vi "Waveform CDB to power level.vi"(11 "Waveform CDB":waveform(cdb)) -> (3 "Power [Watt]":dbl)   [LabVIEW 2020]
uses:
  <vilib>/Analysis/5stat.llb/RMS (DBL).vi
  <vilib>/Analysis/NI_AALPro.lvlib
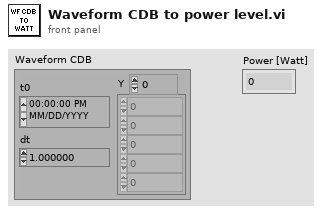
[diagram p1: front panel]
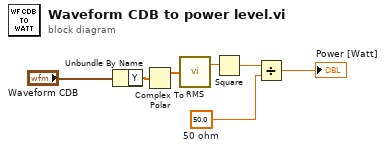
[diagram p0: block diagram]
diagram:
  w7 = 50.0  # 50 ohm
  n1 = Unbundle By Name("Waveform CDB") -> ("Y"=w5:cdb[])
  n2 = Complex To Polar(r * e^(i*theta)=w5) -> (r=w4:dbl[])  [unwired: 1 out]
  n3 = call-poly <vilib>:"RMS.vi"("X"=w4) -> ("rms value"=w3:dbl)  [unwired: 1 out]
  n4 = Square(x=w3) -> (x^2=w2:dbl)
  n5 = Divide(x=w2, y=w7) -> (x/y=→"Power [Watt]":dbl)
